vi "Read Configuration File.vi"(8 "error in (no error)":errorcluster, 11 "Sequence Experiment":refnum<class "Control Experiment.lvclass">) -> (0 "error out":errorcluster, 3 "Sequence Experiment out":refnum<class "Control Experiment.lvclass">)   [LabVIEW 2019, in "Control Experiment.lvclass"]
uses:
  Control Experiment.lvclass
  <userlib>/LevyLab/Instrument Framework/SMOs/Configuration/Configuration.lvclass
  <userlib>/LevyLab/Instrument Framework/SMOs/Instrument/Instrument.lvclass
  C:/Program Files (x86)/National Instruments/LabVIEW 2016/user.lib/LevyLab/Levylab Instruments/SMOs/Instrument/Instrument.lvclass
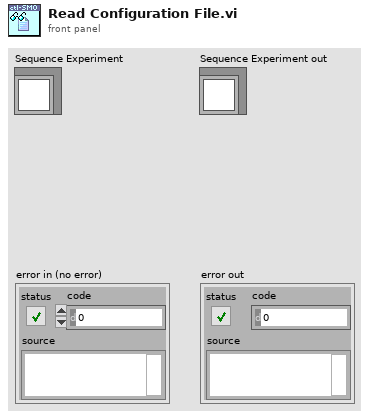
[diagram p1: front panel]
types:
  T1 = typedef "Control Experiment.lvclass/Control Experiment.Configuration--Cluster.ctl" = cluster{"Example Setting 1":dbl, "Example Setting 2":dbl, "Example Setting 3":string}
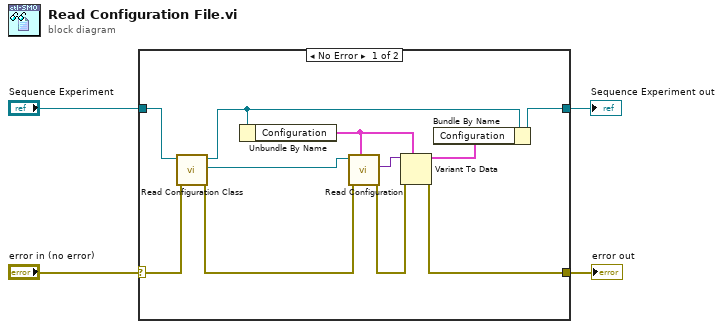
[diagram p0: block diagram]
diagram:
  n1 = case shown="No Error" "error in (no error)" {
    selector: "error in (no error)" -> [w8 w17]
    tunnel: "Sequence Experiment" -> [w11 w16]
    tunnel: [w6 w16] -> w3
    tunnel: [w9 w17] -> w2
    frame No Error {
      n2 = call <userlib>:"Read Configuration Class.vi"("error in (no error)"=w8, "Instrument in"=w11) -> ("error out"=w12:errorcluster, "Configuration"=w13:refnum<class "Configuration.lvclass">, "Instrument out"=w5:refnum<class "Control Experiment.lvclass">)  [unwired: 7 in]
      n3 = Unbundle By Name(w5) -> ("Configuration"=w7:T1)
      n4 = call <userlib>:"Read Configuration.vi"("INI Fomatted Cluster Type"=w7, "error in (no error)"=w12, "Configuration in"=w13) -> ("error out"=w14:errorcluster, "Configuration"=w15:variant)  [unwired: 6 in, 1 out]
      n5 = Variant To Data(error in=w14, type=w7, Variant=w15) -> (data=w10:T1, error out=w9:errorcluster)
      n6 = Bundle By Name(cluster=w5, "Configuration"=w10) -> (w6:refnum<class "Control Experiment.lvclass">)
    }
    frame Error {
    }
  }
  "Sequence Experiment out" <- w3
  "error out" <- w2
